vi "getWaypoints.vi"(8 "Error In":errorcluster, 11 "Idle in":refnum<class "Idle.lvclass">) -> (0 "Error Out":errorcluster, 2 "Waypoint Array":refnum<class "Waypoint.lvclass">[](array[class]), 3 "Idle out":refnum<class "Idle.lvclass">)   [LabVIEW 2013, in "Idle.lvclass"]
uses:
  Idle.lvclass
  Waypoint/Waypoint.lvclass
  GenericMission/GenericMission.lvclass
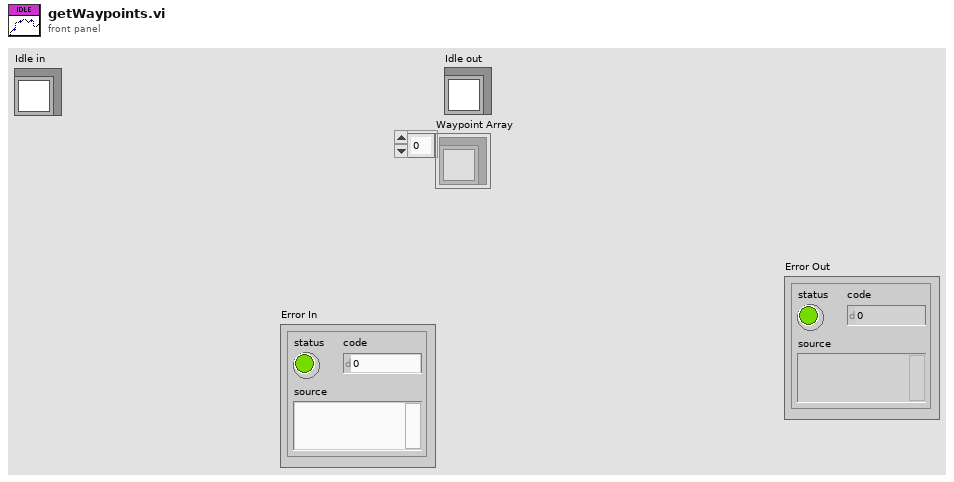
[diagram p1: front panel]
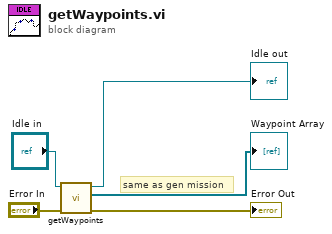
[diagram p0: block diagram]
diagram:
  # "same as gen mission"
  n1 = call-parent "getWaypoints.vi"("Error In"="Error In", "GenericMission in"="Idle in") -> ("Error Out"=→"Error Out":errorcluster, "Waypoint Array"=→"Waypoint Array":refnum<class "Waypoint.lvclass">[], "GenericMission out"=→"Idle out":refnum<class "Idle.lvclass">)  [unwired: 7 in]
